vi "Program_1_Global.vi"() -> ()   [LabVIEW 2024]
panel:
  out "stop":bool
  out "(m, n)":dbl
  out "Max":dbl
  out "Min":dbl
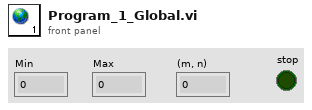
[diagram p1: front panel]
diagram:
